vi "Write PAS.vi"(8 "error in (no error)":errorcluster, 10 "PAS Library.lvlib:PAS Data":refnum<class "PAS Data.lvclass">, 11 "gData in":refnum<class "gData.lvclass">) -> (0 "error out":errorcluster, 3 "gData out":refnum<class "gData.lvclass">)   [LabVIEW 2016, in "gData.lvclass"]
uses:
  gData.lvclass
  <vilib>/MSR Consulting, LLC/General Reuse/PAS/Data/Main/PAS Data.lvclass
  gData.lvclass/gData.ctl
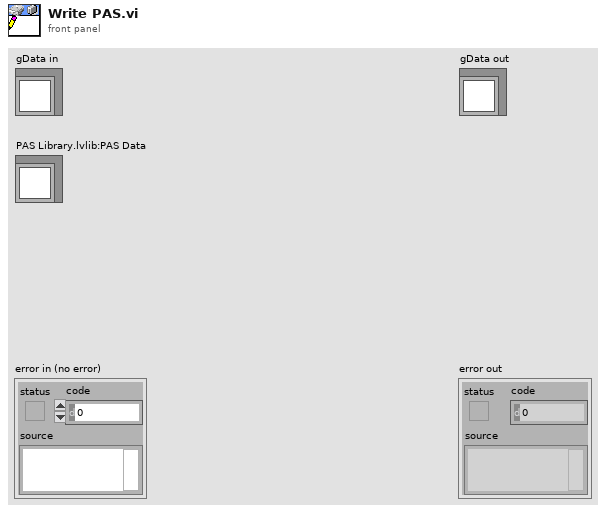
[diagram p1: front panel]
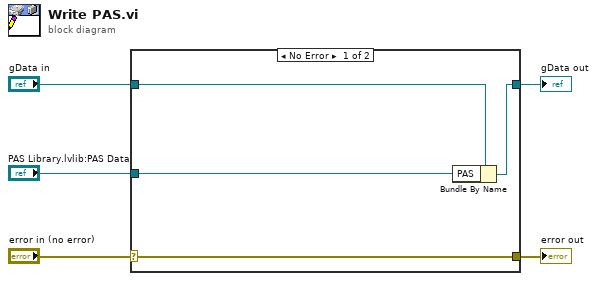
[diagram p0: block diagram]
diagram:
  n1 = case shown="No Error" "error in (no error)" {
    selector: "error in (no error)" -> [w9 w10]
    tunnel: [w9 w10] -> w4
    tunnel: [w7 w11] -> w2
    tunnel: "gData in" -> [w8 w11]
    tunnel: "PAS Library.lvlib:PAS Data" -> [w6 _]
    frame No Error {
      n2 = Bundle By Name(cluster=w8, "PAS"=w6) -> (w7:refnum<class "gData.lvclass">)
    }
    frame Error {
    }
  }
  "error out" <- w4
  "gData out" <- w2
